vi "omega_sub_Encoder_800ppr.vi"(5 "mt0":u32, 7 "omega_pre":fxp<+/-,36,13>, 8 "ticks_m_pre":u32, 9 "ticks":u32, 10 "count_pre":i32, 11 "count":i32) -> (0 "ticks_m":u32, 1 "mt":u32, 3 "omega":fxp<+/-,36,13>)   [LabVIEW 2014]
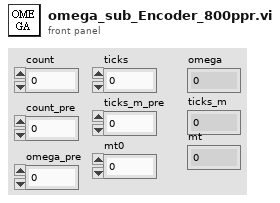
[diagram p1: front panel]
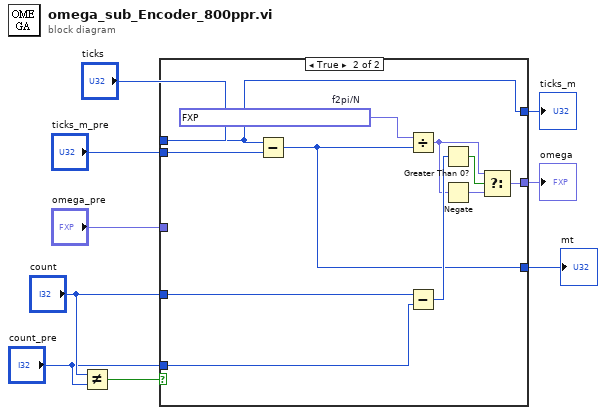
[diagram p0: block diagram]
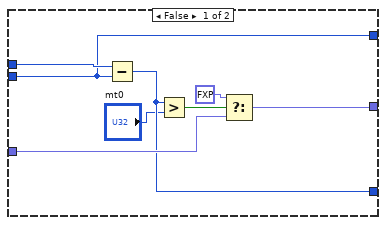
[diagram p2: hidden frame]
diagram:
  n1 = Not Equal?(x="count", y="count_pre") -> (x != y?=w9:bool)
  n2 = case shown="True" w9 {
    tunnel: "ticks" -> [w17 w25]
    tunnel: "count" -> [_ w28]
    tunnel: "count_pre" -> [_ w27]
    tunnel: [w16 w25] -> w2
    tunnel: "ticks_m_pre" -> [w16 w24]
    tunnel: [w13 w20] -> w6
    tunnel: "omega_pre" -> [w14 _]
    tunnel: [w11 w19] -> w1
    frame False {
      n3 = Subtract(x=w17, y=w16) -> (x-y=w11:u32)
      n4 = Greater?(x=w11, y="mt0") -> (0:w15:bool)
      n5 = Select(t=fxp<+/-,20,9> 0.0, s=w15, f=w14) -> (s? t:f=w13:fxp<+/-,36,13>)
    }
    frame True {
      w18 = fxp<+,40,19> 314159.26535892487  # f2pi/N
      n6 = Subtract(x=w25, y=w24) -> (x-y=w19:u32)
      n7 = Divide(x=w18, y=w19) -> (x/y=w22:fxp<+/-,36,13>)
      n8 = Subtract(x=w28, y=w27) -> (x-y=w26:i32)
      n9 = Greater Than 0?(x=w26) -> (x > 0?=w21:bool)
      n10 = Negate(x=w22) -> (-x=w23:fxp<+/-,36,13>)
      n11 = Select(t=w22, s=w21, f=w23) -> (s? t:f=w20:fxp<+/-,36,13>)
    }
  }
  "omega" <- w6
  "ticks_m" <- w2
  "mt" <- w1
